vi "Register Values to String.vi"(0 "Register Values":u16[](array[numeric]) caption="寄存器值", 3 "Register Number":dbl=1.0 caption="寄存器数量" min=1.0) -> (6 "String Out":string caption="输出字符串")   [LabVIEW 2023, in "Longer Pump dLSP501 Series.lvlib"]
uses:
  <instrlib>/Longer Pump dLSP501 Modbus RTU Series/Longer Pump dLSP501 Series.lvlib
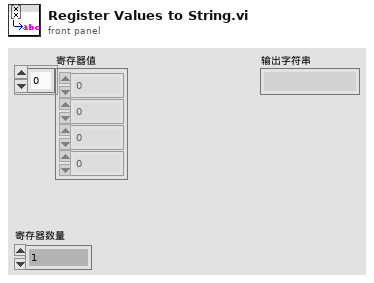
[diagram p1: front panel]
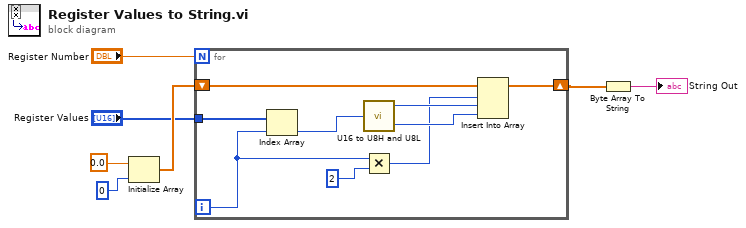
[diagram p0: block diagram]
diagram:
  n1 = Initialize Array(0.0 ("元素"), 0 ("维数大小")) -> (w7:dbl[])
  n2 = for {
    N: "Register Number" -> [_]
    shift-right: [w14] -> w3
    shift-left: w7 -> [w15]
    tunnel: "Register Values" -> [w8]
    i -> [w11]
    n3 = Index Array(array=w8, index=w11) -> (element=w16:u16)
    n4 = call <instrlib>:"U16 to U8H and U8L.vi"("U16"=w16) -> ("Lower Byte"=w13:u8, "Higher Byte"=w12:u8)  [unwired: 3 in]
    n5 = Multiply(x=w11, y=2 ("x")) -> (x*y=w10:i32)
    n6 = Insert Into Array(array=w15, index=w10, new element #1=w12, new element #2=w13) -> (w14:dbl[])
  }
  n7 = Byte Array To String(unsigned byte array=w3) -> (string=→"String Out":string)
